vi "题目 2.vi"() -> ()   [LabVIEW 2017]
panel:
  in  "digital waveform":digitalwaveform(waveform) caption="数字波形"
  out "数字波形图":digitalwaveform(graph)
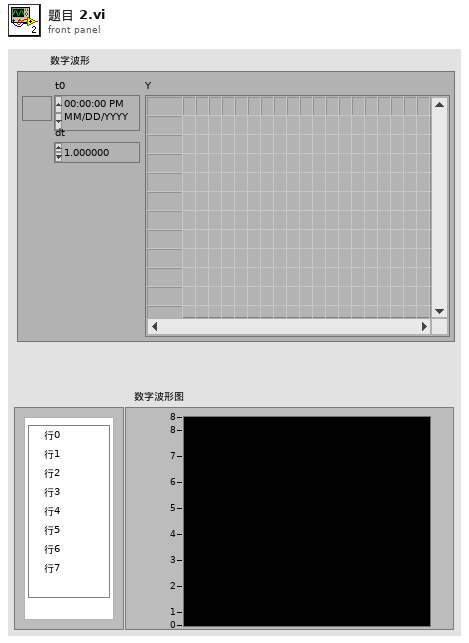
[diagram p1: front panel]
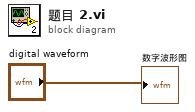
[diagram p0: block diagram]
diagram:
  "数字波形图" <- "digital waveform"
